vi "AI Post Step.vi"(8 "error in (no error)":errorcluster, 9 "AIRead":T1, 10 "Socket No":u16=1, 11 "AI in":refnum<class "AI.lvclass">) -> (0 "error out":errorcluster, 1 "AnalogRead":dbl[](array[numeric]), 2 "Report Text":string, 3 "AI out":refnum<class "AI.lvclass">, 4 "Selected Physical Channel":string[](array[string]))   [LabVIEW 2023, in "HardwareAbstractionLayer_LVOOP.lvlib" / "AI.lvclass"]
uses:
  AI.lvclass
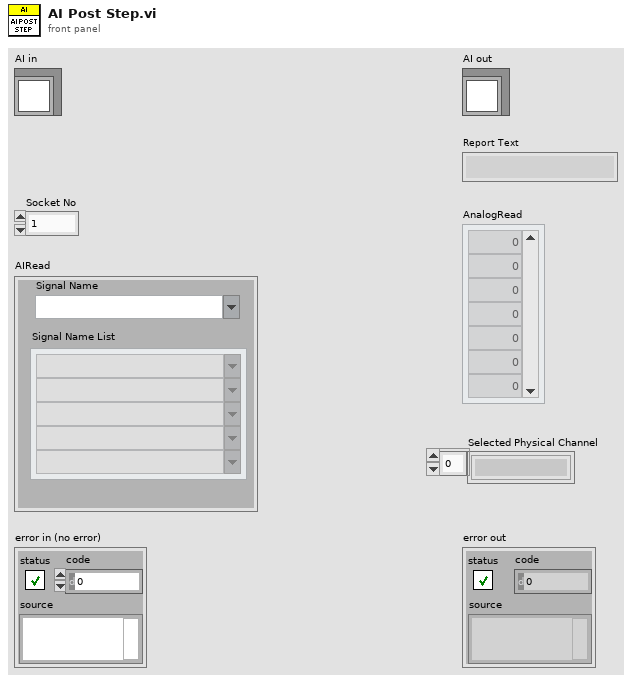
[diagram p1: front panel]
types:
  T1 = cluster{"Signal Name":string, "Signal Name List":string[]}
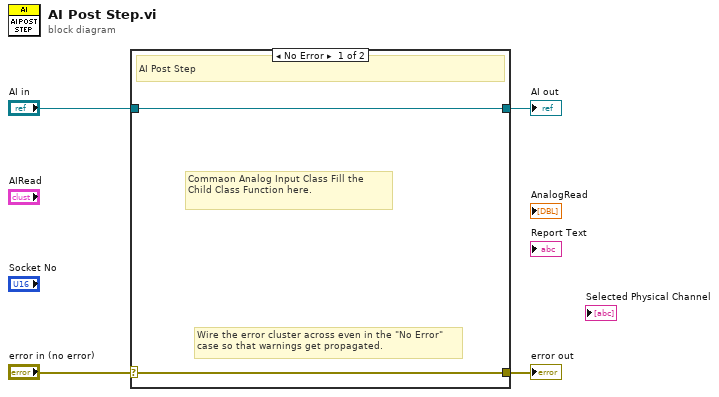
[diagram p0: block diagram]
diagram:
  n1 = case shown="No Error" "error in (no error)" {
    selector: "error in (no error)" -> [w5 w8]
    tunnel: [w5 w8] -> w3
    tunnel: [w6 w7] -> w1
    tunnel: "AI in" -> [w6 w7]
    frame No Error {
      # "Wire the error cluster across even in the \"No Error\"\ncase so that warnings get propagated."
      # "Commaon Analog Input Class Fill the Child Class Function here."
      # "AI Post Step"
    }
    frame Error {
    }
  }
  "error out" <- w3
  "AI out" <- w1
